vi "temperature_controller.vi"() -> ()   [LabVIEW 2017]
panel:
  out "Waveform Graph":dbl[](graph)
  out "Waveform Chart":dbl(graph)
  in  "stop":bool
  out "Temp Value (C)":dbl
  out "?":dbl
  in  "Temperature (F)":dbl(slide) scale=0.0..200.0
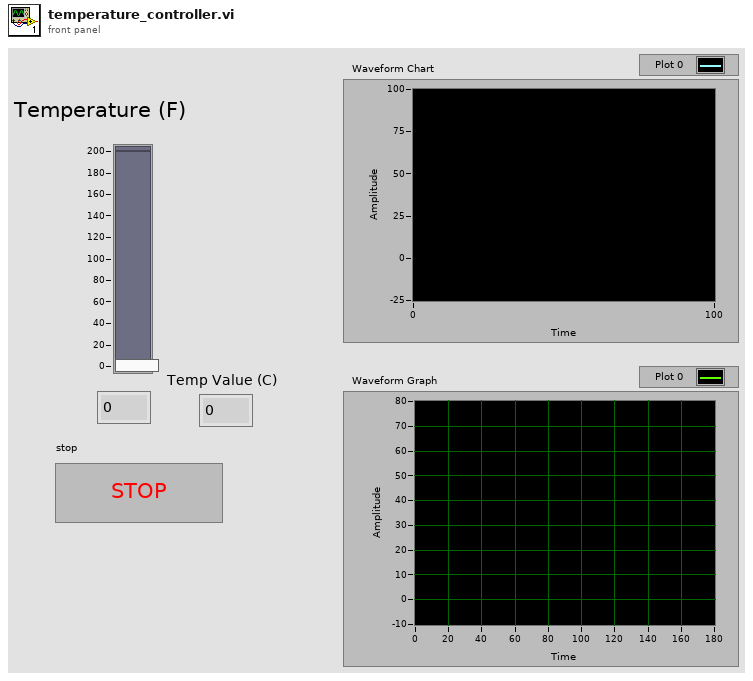
[diagram p1: front panel]
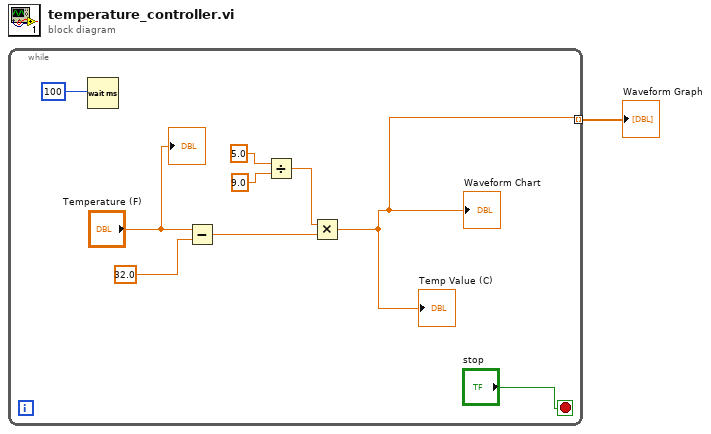
[diagram p0: block diagram]
diagram:
  n1 = while {
    tunnel: [w2] -> w1 mode=indexing
    stop <- "stop" stop-if-true
    n2 = Wait (ms)(milliseconds to wait=100) -> ()  [unwired: 1 out]
    n3 = Subtract(x="Temperature (F)", y=32.0) -> (x-y=w9:dbl)
    n4 = Divide(x=5.0, y=9.0) -> (x/y=w6:dbl)
    n5 = Multiply(x=w6, y=w9) -> (x*y=w2:dbl)
    "Temp Value (C)" <- w2
    "Waveform Chart" <- w2
    "?" <- "Temperature (F)"
  }
  "Waveform Graph" <- w1
